vi "LSX Get DLL Version String.vi"(8 "error in (no error)":errorcluster, 9 "lMaxLen":i32, 10 "pcVers":string, 11 "lLSID":i32) -> (0 "error out":errorcluster, 2 "pcVers out":string, 3 "function return":i32)   [LabVIEW 2018, in "Tango.lvlib"]
doc: "TANGOAPI int TANGOCALL LSX_GetDLLVersionString (int lLSID, char *pcVers, int lMaxLen);"
uses:
  <userlib>/Tango/Tango.lvlib
  <userlib>/Tango/Tango_DLL.dll
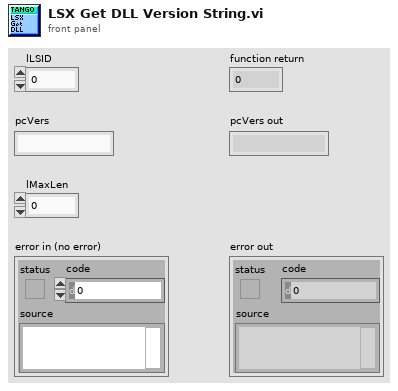
[diagram p1: front panel]
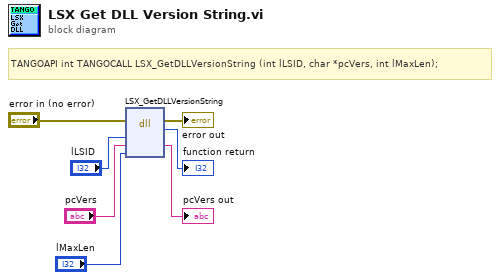
[diagram p0: block diagram]
diagram:
  # "TANGOAPI int TANGOCALL LSX_GetDLLVersionString (int lLSID, char *pcVers, int lMaxLen);"
  n1 = dll-call lib="C:/Program Files (x86)/National Instruments/LabVIEW 2018/user.lib/Tango/Tango_DLL.*" fn="LSX_GetDLLVersionString"(error in="error in (no error)", "lLSID"="lLSID", "pcVers"="pcVers", "lMaxLen"="lMaxLen") -> (error out=→"error out":errorcluster, →"function return":i32, "pcVers"=→"pcVers out":string)  [unwired: 4 in, 1 out]
